vi "Parse Version.vi"(8 "error in":errorcluster, 11 "Node In":refnum<k20>) -> (0 "error out":errorcluster, 2 "Version":string, 3 "Node Out":refnum<k20>)   [LabVIEW 2024, in "Parser.lvlib" / "Custom Device Config.lvclass"]
uses:
  Custom Device Config.lvclass
  <vilib>/xml/NI_XML.lvlib
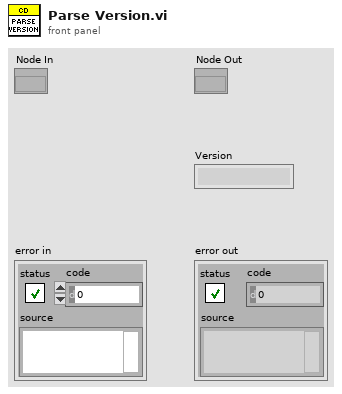
[diagram p1: front panel]
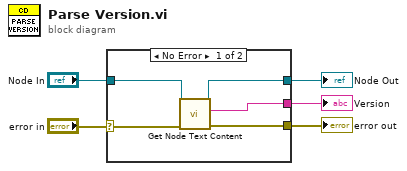
[diagram p0: block diagram]
diagram:
  n1 = case shown="No Error" "error in" {
    selector: "error in" -> [w9 w12]
    tunnel: [w10 w12] -> w4
    tunnel: "Node In" -> [w7 w11]
    tunnel: [w6 w11] -> w2
    tunnel: [w8 _] -> w1
    frame No Error {
      n2 = call <vilib>:"Get Node Text Content.vi"("error in (no error)"=w9, "node in"=w7) -> ("error out"=w10:errorcluster, "node text"=w8:string, "node out"=w6:refnum<k20>)  [unwired: 7 in]
    }
    frame Error {
    }
  }
  "Node Out" <- w2
  "error out" <- w4
  "Version" <- w1
